vi "StopCursorOscilloscopeMoving.vi"(8 "error in (no error)":errorcluster, 10 "Boolean":bool, 11 "Control-Client in":refnum<class "Control-Client.lvclass">) -> (0 "error out":errorcluster, 3 "Control-Client out":refnum<class "Control-Client.lvclass">)   [LabVIEW 2015, in "Control-Client.lvclass"]
uses:
  Control-Client.lvclass
  Control-Client.lvclass/Control-Client.ctl
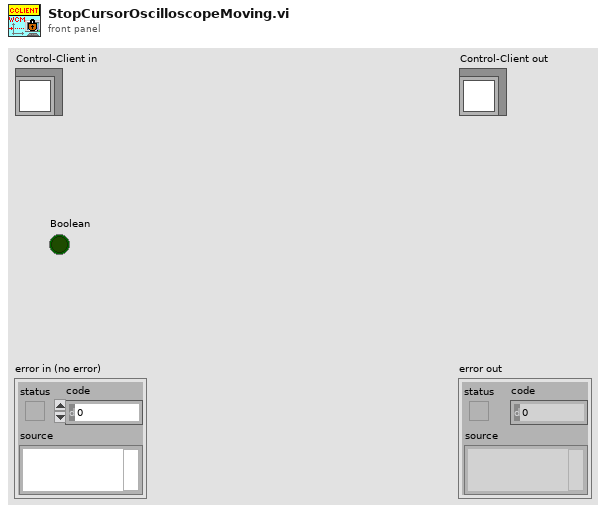
[diagram p1: front panel]
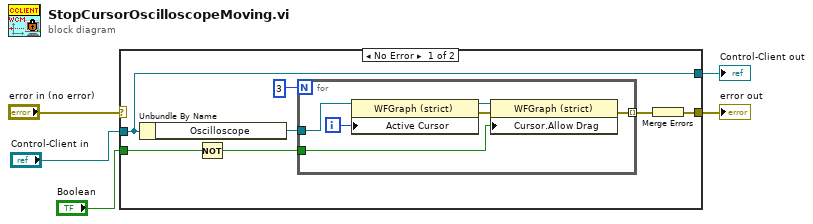
[diagram p0: block diagram]
diagram:
  n1 = case shown="No Error" "error in (no error)" {
    selector: "error in (no error)" -> [_ w20]
    tunnel: [w7 w20] -> w4
    tunnel: [w12 w19] -> w2
    tunnel: "Control-Client in" -> [w12 w19]
    tunnel: "Boolean" -> [w11 _]
    frame No Error {
      n2 = Unbundle By Name(w12) -> ("Oscilloscope"=w9:refnum<vi>)
      n3 = Not(x=w11) -> (.not. x?=w6:bool)
      n4 = for {
        N: 3 -> [_]
        tunnel: w9 -> [w16]
        tunnel: [w14] -> w8 mode=indexing
        tunnel: w6 -> [w13]
        i -> [w15]
        n5 = property class="WFGraph (strict)"(reference=w16, "Active Cursor"=w15) -> (reference out=w18:refnum<vi>, error out=w17:errorcluster)  [unwired: 1 in]
        n6 = property class="WFGraph (strict)"(reference=w18, error in=w17, "Cursor.Allow Drag"=w13) -> (error out=w14:errorcluster)  [unwired: 1 out]
      }
      n7 = Merge Errors(w8) -> (w7:errorcluster)
    }
    frame Error {
    }
  }
  "error out" <- w4
  "Control-Client out" <- w2
